vi "ReadPMUData_RT.vi"(1 "I_BAT2":fxp<+/-,20,5> format="%#_17g", 4 "I_BAT1":fxp<+,20,5> format="%#_17g", 5 "V_BAT2":fxp<+,20,5> format="%#_17g", 6 "I_PV2":fxp<+/-,20,5> format="%#_17g", 7 "V_PV2":fxp<+/-,20,5> format="%#_17g", 8 "V_BAT1":fxp<+/-,20,5> format="%#_17g", 9 "I_PV1":fxp<+,20,5> format="%#_17g", 10 "V_PV1":fxp<+,20,5> format="%#_17g") -> (2 "measurements":T1)   [LabVIEW 2021]
uses:
  acdc-PV-emulators/General Purpose/references.ctl
panel:
  in  "I ratio":dbl=40.0
  in  "V ratio":dbl=100.0
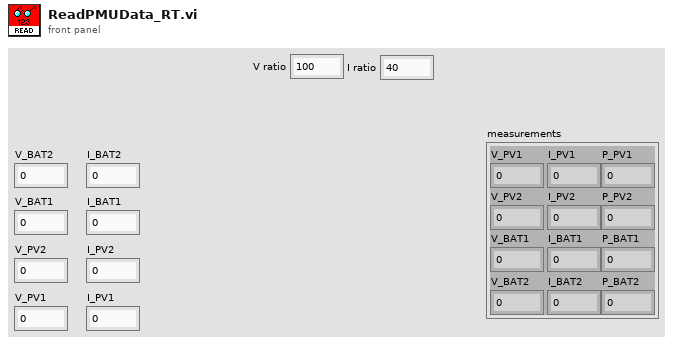
[diagram p1: front panel]
types:
  T1 = cluster{"V_PV1":dbl, "I_PV1":dbl, "V_PV2":dbl, "I_PV2":dbl, "P_PV2":dbl, "V_BAT1":dbl, "I_BAT1":dbl, "P_BAT1":dbl, "V_BAT2":dbl, "I_BAT2":dbl, "P_BAT2":dbl, "P_PV1":dbl}
  T2 = typedef "references.ctl" = cluster{"P1":dbl, "\nP2":dbl, "P3":dbl, "P4":dbl, "VSC":dbl, "PSC":dbl}
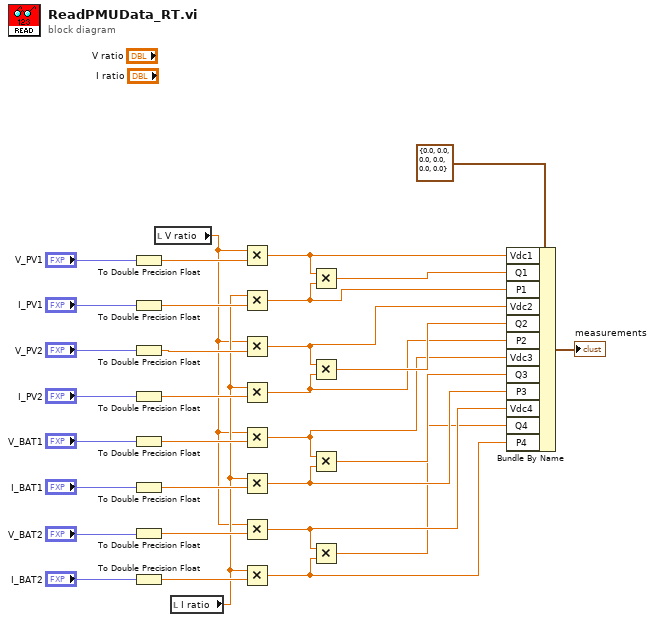
[diagram p0: block diagram]
diagram:
  n1 = To Double Precision Float(number="V_PV1") -> (double precision float=w24:dbl)
  n2 = To Double Precision Float(number="I_PV1") -> (double precision float=w23:dbl)
  n3 = To Double Precision Float(number="V_PV2") -> (double precision float=w22:dbl)
  n4 = To Double Precision Float(number="I_PV2") -> (double precision float=w21:dbl)
  n5 = To Double Precision Float(number="V_BAT1") -> (double precision float=w20:dbl)
  n6 = To Double Precision Float(number="I_BAT1") -> (double precision float=w25:dbl)
  n7 = To Double Precision Float(number="V_BAT2") -> (double precision float=w26:dbl)
  n8 = To Double Precision Float(number="I_BAT2") -> (double precision float=w27:dbl)
  n9 = local read "V ratio"() -> (w15:dbl)
  n10 = local read "I ratio"() -> (w16:dbl)
  n11 = Multiply(x=w15, y=w24) -> (x*y=w14:dbl)
  n12 = Multiply(x=w16, y=w23) -> (x*y=w12:dbl)
  n13 = Multiply(x=w15, y=w22) -> (x*y=w11:dbl)
  n14 = Multiply(x=w16, y=w21) -> (x*y=w9:dbl)
  n15 = Multiply(x=w15, y=w20) -> (x*y=w8:dbl)
  n16 = Multiply(x=w16, y=w25) -> (x*y=w6:dbl)
  n17 = Multiply(x=w15, y=w26) -> (x*y=w5:dbl)
  n18 = Multiply(x=w16, y=w27) -> (x*y=w3:dbl)
  n19 = Multiply(x=w14, y=w12) -> (x*y=w13:dbl)
  n20 = Multiply(x=w11, y=w9) -> (x*y=w10:dbl)
  n21 = Multiply(x=w8, y=w6) -> (x*y=w7:dbl)
  n22 = Multiply(x=w5, y=w3) -> (x*y=w4:dbl)
  n23 = Bundle By Name(cluster=T2 {"P1"=0.0, "\nP2"=0.0, "P3"=0.0, "P4"=0.0, "VSC"=0.0, "PSC"=0.0} ("Meas"), "Vdc1"=w14, "Q1"=w13, "P1"=w12, "Vdc2"=w11, "Q2"=w10, "P2"=w9, "Vdc3"=w8, "Q3"=w7, "P3"=w6, "Vdc4"=w5, "Q4"=w4, "P4"=w3) -> (→"measurements":T2)
